vi "Ventas update or create.vi"(8 "error in (no error)":errorcluster, 9 "i":i32, 10 "Full pedido":string[][](array[string]), 11 "Vendidos":i32) -> (0 "error out":errorcluster)   [LabVIEW 2018]
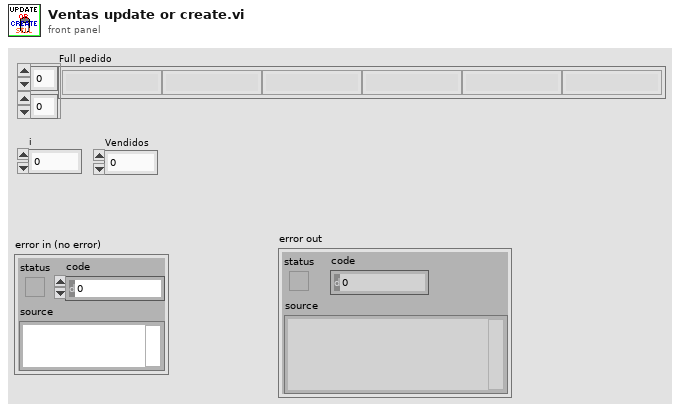
[diagram p1: front panel]
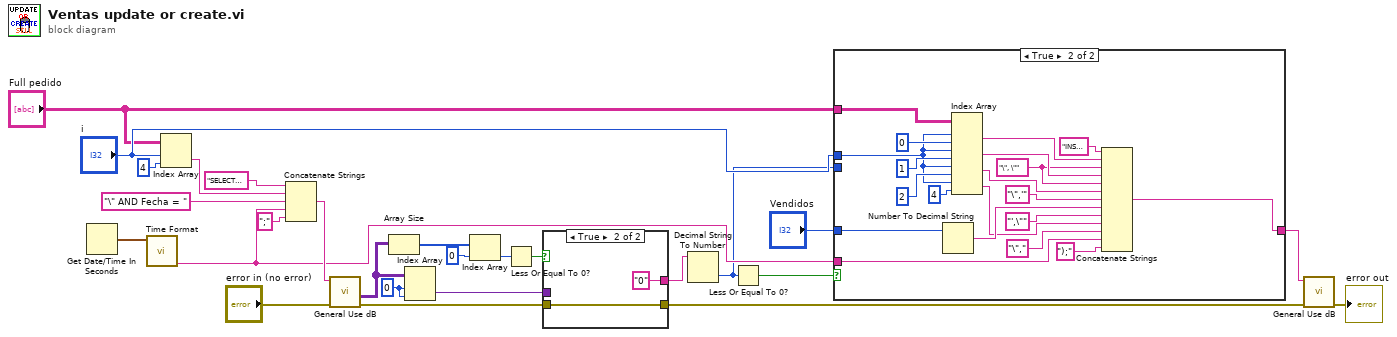
[diagram p0: block diagram]
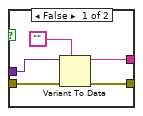
[diagram p2: hidden frame]
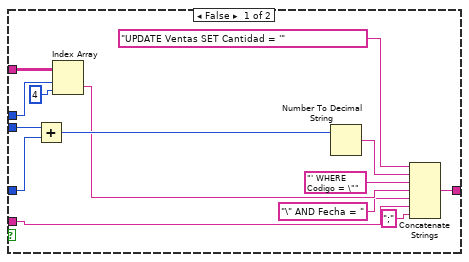
[diagram p3: hidden frame]
diagram:
  w23 = 0 ("index (col)")
  n1 = Get Date/Time In Seconds() -> (seconds since 1Jan1904=w7:timestamp)
  n2 = call "Time Format.vi"("time stamp"=w7) -> ("concatenated string"=w13:string)  [unwired: 10 in]
  n3 = Index Array(array="Full pedido", index (row)="i", index (col)=4) -> (element=w17:string)
  n4 = Concatenate Strings("SELECT Cantidad FROM Ventas WHERE Codigo =\"", w17, "\" AND Fecha = " ("string"), w13, ";" ("string")) -> (w25:string)
  n5 = call "General Use dB.vi"("error in (no error)"="error in (no error)", "Query"=w25) -> ("error out"=w22:errorcluster, "Return Data"=w6:variant[][])  [unwired: 8 in]
  n6 = Array Size(array=w6) -> (size(s)=w5:i32[])
  n7 = Index Array(array=w6, index (row)=w23, index (col)=w23) -> (element=w21:variant)
  n8 = Index Array(array=w5, index=0) -> (element=w3:i32)
  n9 = Less Or Equal To 0?(x=w3) -> (x <= 0?=w2:bool)
  n10 = case shown="True" w2 {
    tunnel: w22 -> [w31 w32]
    tunnel: w21 -> [w30 _]
    tunnel: [w28 "0"] -> w20
    tunnel: [w27 w32] -> w9
    frame False {
      n11 = Variant To Data(error in=w31, type="", Variant=w30) -> (data=w28:string, error out=w27:errorcluster)
    }
    frame True {
    }
  }
  n12 = Decimal String To Number(string=w20) -> (number=w11:i32)  [unwired: 2 in, 1 out]
  n13 = Less Or Equal To 0?(x=w11) -> (x <= 0?=w19:bool)
  n14 = case shown="True" w19 {
    tunnel: "i" -> [w39 w62]
    tunnel: "Full pedido" -> [w38 w63]
    tunnel: "Vendidos" -> [w44 w54]
    tunnel: w13 -> [w35 w49]
    tunnel: [w41 w53] -> w10
    tunnel: w11 -> [w45 _]
    frame False {
      n15 = Add(x=w45, y=w44) -> (x+y=w43:i32)
      n16 = Index Array(array=w38, index (row)=w39, index (col)=4) -> (element=w37:string)
      n17 = Number To Decimal String(number=w43) -> (decimal integer string=w42:string)  [unwired: 1 in]
      n18 = Concatenate Strings("UPDATE Ventas SET Cantidad = '", w42, "' WHERE Codigo = \"" ("string"), w37, "\" AND Fecha = " ("string"), w35, ";" ("string")) -> (w41:string)
    }
    frame True {
      w58 = "\", \"" ("string")
      n19 = Number To Decimal String(number=w54) -> (decimal integer string=w55:string)  [unwired: 1 in]
      n20 = Index Array(array=w63, index (row) #1=w62, index (col) #1=0 ("disabled index (col)"), index (row) #2=w62, index (col) #2=1 ("disabled index (col)"), index (row) #3=w62, index (col) #3=2 ("disabled index (col)"), index (row) #4=w62, index (col) #4=4 ("disabled index (col)")) -> (element #1=w60:string, element #2=w59:string, element #3=w57:string, element #4=w51:string)
      n21 = Concatenate Strings("INSERT INTO Ventas (Modelo, Color, Talla, Cantidad, Codigo, Fecha) Values (\"", w60, w58, w59, w58, w57, "\",'" ("string"), w55, "',\"" ("string"), w51, "\"," ("string"), w49, ");" ("string")) -> (w53:string)
    }
  }
  n22 = call "General Use dB.vi"("error in (no error)"=w9, "Query"=w10) -> ("error out"=→"error out":errorcluster)  [unwired: 8 in, 1 out]
